vi "Get Firmware Program Interfaces.vi"(8 "Error In":errorcluster, 10 "Device Index":i32, 11 "Family Index":i32) -> (0 "Error Out":errorcluster, 3 "Firmware Program Interfaces":string[](array[string]))   [LabVIEW 2019, in "LMH-LINX.lvlib"]
uses:
  <vilib>/MakerHub/LINX/LMH-LINX.lvlib
  <vilib>/MakerHub/LINX/Private/Type Defs/All Firmware Data FGV States.ctl
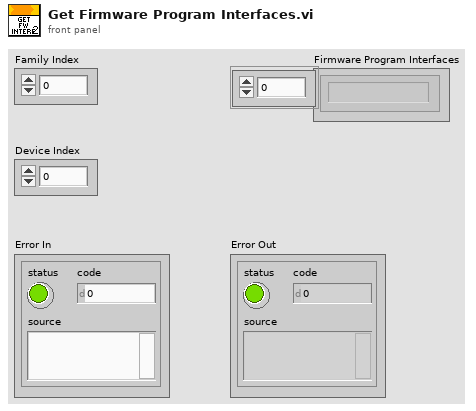
[diagram p1: front panel]
types:
  T1 = typedef "LMH-LINX.lvlib/All Firmware Data FGV States.ctl" = enum16{"Set", "Get"}
  T2 = typedef "LMH-LINX.lvlib/Device Data.ctl" = cluster{"Family ID":i32, "Family Name":string, "Device ID":i32, "Device Name":string, "Firmware Program Interfaces":string[], "Path":path}
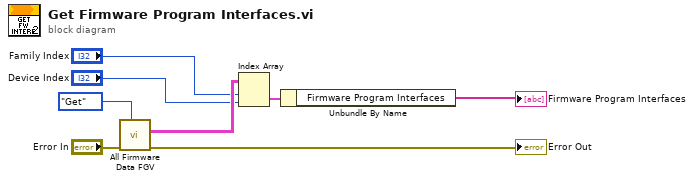
[diagram p0: block diagram]
diagram:
  n1 = call <vilib>:"All Firmware Data FGV.vi"("All Firmware Data FGV States"=All_Firmware_Data_FGV_States."Get", "Error In"="Error In") -> ("Error Out"=→"Error Out":errorcluster, "Devices"=w6:T2[][])  [unwired: 6 in, 2 out]
  n2 = Index Array(array=w6, index (row)="Family Index", index (col)="Device Index") -> (element=w3:T2)
  n3 = Unbundle By Name(w3) -> ("Firmware Program Interfaces"=→"Firmware Program Interfaces":string[])
